vi "Tournament String to Data.vi"(11 "Tournament Data String":string) -> (2 "Tournament Data Array":T1(array[cluster]), 3 "Tournament Player Name Array":string[](array[string]))   [LabVIEW 2021]
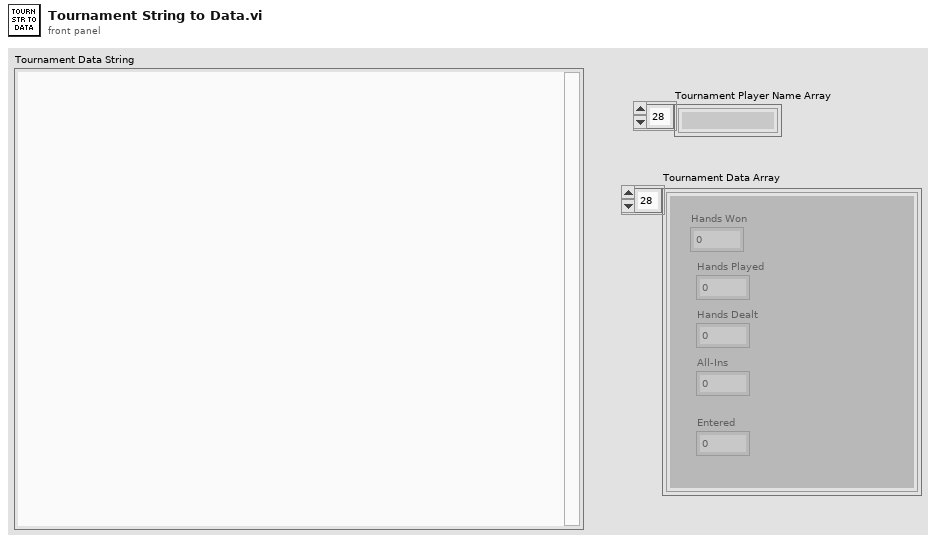
[diagram p1: front panel]
types:
  T1 = cluster{"Hands Won":u32, "Hands Played":u32, "Hands Dealt":u32, "All-Ins":u32, "Entered":u32}[]
  T2 = cluster{"Numeric":i32, "Numeric":i32, "Numeric":i32, "Numeric":i32, "Numeric":i32}
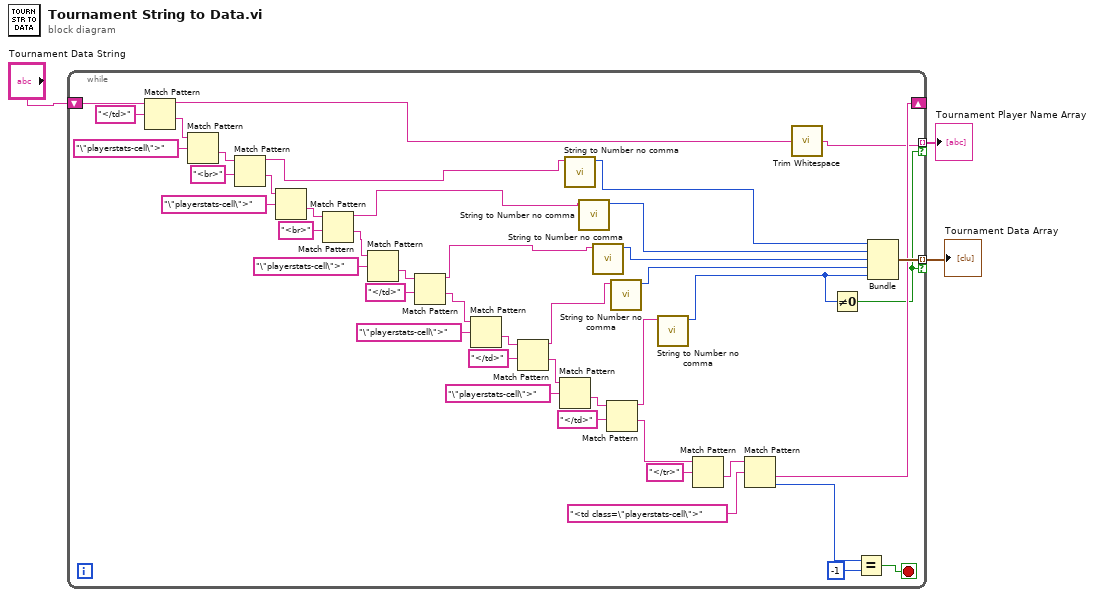
[diagram p0: block diagram]
diagram:
  n1 = while {
    shift-right: [w8] -> _
    shift-left: "Tournament Data String" -> [w47]
    tunnel: [w5] -> w2 mode=indexing if=w6
    tunnel: [w22] -> w1 mode=indexing if=w6
    stop <- w23 stop-if-true
    n2 = Match Pattern(string=w47, regular expression="</td>") -> (before substring=w4:string, after substring=w45:string)  [unwired: 1 in, 2 out]
    n3 = Match Pattern(string=w45, regular expression="\"playerstats-cell\">") -> (after substring=w43:string)  [unwired: 1 in, 3 out]
    n4 = Match Pattern(string=w43, regular expression="<br>") -> (before substring=w21:string, after substring=w38:string)  [unwired: 1 in, 2 out]
    n5 = Match Pattern(string=w38, regular expression="\"playerstats-cell\">") -> (after substring=w40:string)  [unwired: 1 in, 3 out]
    n6 = Match Pattern(string=w40, regular expression="<br>") -> (before substring=w19:string, after substring=w35:string)  [unwired: 1 in, 2 out]
    n7 = Match Pattern(string=w35, regular expression="\"playerstats-cell\">") -> (after substring=w37:string)  [unwired: 1 in, 3 out]
    n8 = Match Pattern(string=w37, regular expression="</td>") -> (before substring=w17:string, after substring=w30:string)  [unwired: 1 in, 2 out]
    n9 = Match Pattern(string=w30, regular expression="\"playerstats-cell\">") -> (after substring=w31:string)  [unwired: 1 in, 3 out]
    n10 = Match Pattern(string=w31, regular expression="</td>") -> (before substring=w15:string, after substring=w26:string)  [unwired: 1 in, 2 out]
    n11 = Match Pattern(string=w26, regular expression="\"playerstats-cell\">") -> (after substring=w29:string)  [unwired: 1 in, 3 out]
    n12 = call "String to Number no comma.vi"("Number String"=w21) -> ("Numeric"=w20:i32)  [unwired: 10 in]
    n13 = call "String to Number no comma.vi"("Number String"=w19) -> ("Numeric"=w18:i32)  [unwired: 10 in]
    n14 = call "String to Number no comma.vi"("Number String"=w17) -> ("Numeric"=w16:i32)  [unwired: 10 in]
    n15 = Match Pattern(string=w29, regular expression="</td>") -> (before substring=w13:string, after substring=w25:string)  [unwired: 1 in, 2 out]
    n16 = call "String to Number no comma.vi"("Number String"=w15) -> ("Numeric"=w14:i32)  [unwired: 10 in]
    n17 = call "String to Number no comma.vi"("Number String"=w13) -> ("Numeric"=w7:i32)  [unwired: 10 in]
    n18 = Match Pattern(string=w25, regular expression="</tr>") -> (after substring=w11:string)  [unwired: 1 in, 3 out]
    n19 = Match Pattern(string=w11, regular expression="<td class=\"playerstats-cell\">") -> (after substring=w8:string, offset past match=w9:i32)  [unwired: 1 in, 2 out]
    n20 = call <vilib>:"Trim Whitespace.vi"("string"=w4) -> ("trimmed string"=w5:string)  [unwired: 1 in]
    n21 = Not Equal To 0?(x=w7) -> (x != 0?=w6:bool)
    n22 = Equal?(x=w9, y=-1) -> (x = y?=w23:bool)
    n23 = Bundle("Numeric"=w20, "Numeric"=w18, "Numeric"=w16, "Numeric"=w14, "Numeric"=w7) -> (w22:T2)  [unwired: 1 in]
  }
  "Tournament Player Name Array" <- w2
  "Tournament Data Array" <- w1
